vi "mongo_client.vi"(9 "port":i32, 10 "host":string, 11 "conn in":T1) -> (0 "error out":errorcluster)   [LabVIEW 2013]
uses:
  mongo.ctl
panel:
  out "conn out":T1
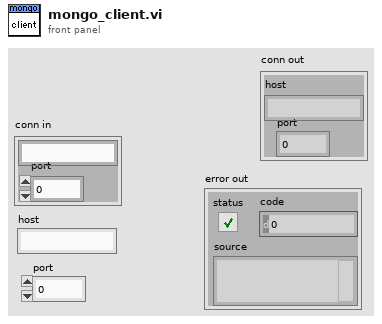
[diagram p1: front panel]
types:
  T1 = typedef "mongo.ctl" = cluster{"host":string, "port":i32}
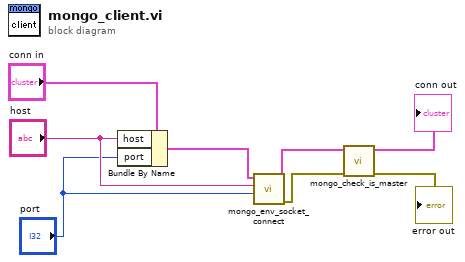
[diagram p0: block diagram]
diagram:
  n1 = Bundle By Name(cluster="conn in", "host"="host", "port"="port") -> (w7:T1)
  n2 = call "mongo_env_socket_connect.vi"("port"="port", "host"="host", "conn in"=w7) -> ("error out"=w6:errorcluster, "conn out"=w3:T1)  [unwired: 7 in]
  n3 = call "mongo_check_is_master.vi"("error in (no error)"=w6, "conn in"=w3) -> ("error out"=→"error out":errorcluster, "conn out"=→"conn out":T1)  [unwired: 8 in]
